vi "Yokogawa GS200 Coarse V ramp.vi"(5 "Time Interval (sec)":dbl=0.5 min=0.1 step=0.1, 6 "stop":bool, 7 "Sweep Time (H:M:S)":dbl=3600.0 format="%<%H:%M:%S>t", 8 "Mapping":bool, 9 "End Voltage (V)":dbl=1e-10 format="%.3e", 10 "Start Voltage (V)":dbl=1e-06 format="%.3e", 11 "Yokogawa GS200 Address":refnum<visa-resource-name>) -> (1 "Last Sent Value":dbl=1e-06 format="%.3e")   [LabVIEW 2020]
uses:
  Global Variables/Voltage Yokogawa Coarse.vi
panel:
  out "Iteration":i32
  out "Prepared Value":dbl=1e-06 format="%.3e"
  # "Add two extra sec for timing."
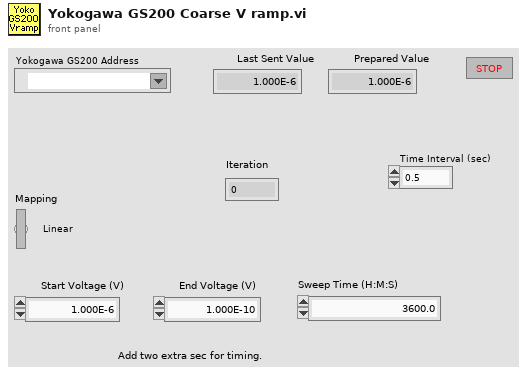
[diagram p1: front panel]
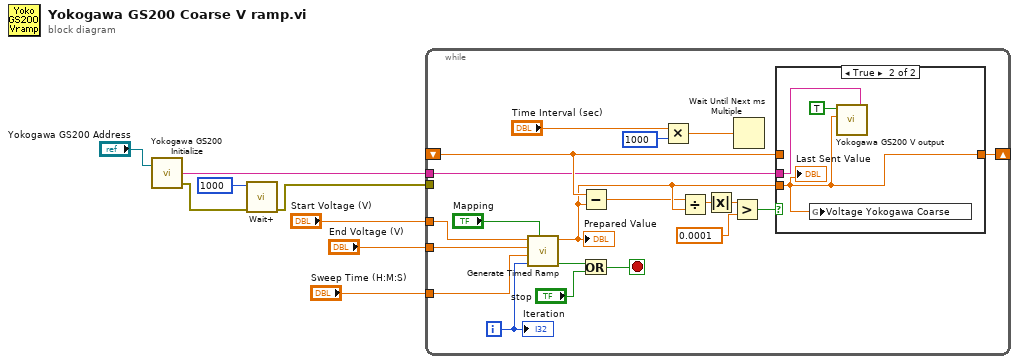
[diagram p0: block diagram]
diagram:
  n1 = call "Yokogawa GS200 Initialize.vi"("VISA resource name"="Yokogawa GS200 Address") -> ("Instrument ID String"=w8:string, "Error Out"=w4:errorcluster)  [unwired: 1 in, 1 out]
  n2 = call "Wait+.vi"("Error In"=w4, "milliseconds to wait"=u32 1000) -> ("Error Out"=w6:errorcluster)  [unwired: 4 in, 1 out]
  n3 = while {
    tunnel: "Start Voltage (V)" -> [w28]
    tunnel: "End Voltage (V)" -> [w27]
    tunnel: "Sweep Time (H:M:S)" -> [w26]
    shift-right: [w19] -> _
    shift-left: _ -> [w17]
    tunnel: w8 -> [w15]
    tunnel: w6 -> [_]
    i -> [w25]
    stop <- w23 stop-if-true
    n4 = call "Generate Timed Ramp.vi"("Log"="Mapping", "Point #"=w25, "Time (Hr:Min:Sec)"=w26, "Stop"=w27, "Start"=w28) -> ("Stop"=w22:bool, "Output"=w16:dbl)  [unwired: 2 out]
    "Prepared Value" <- w16
    n5 = Subtract(x=w17, y=w16) -> (x-y=w11:dbl)
    n6 = Or(x=w22, y="stop") -> (x .or. y?=w23:bool)
    n7 = Multiply(x="Time Interval (sec)", y=u32 1000 ("millisecond multiple")) -> (x*y=w13:dbl)
    n8 = Divide(x=w11, y=w16) -> (x/y=w9:dbl)
    n9 = Absolute Value(x=w9) -> (abs(x)=w10:dbl)
    n10 = Greater?(x=w10, y=0.0001) -> (0:w18:bool)
    n11 = Wait Until Next ms Multiple(millisecond multiple=w13) -> ()  [unwired: 1 out]
    n12 = case shown="True" w18 {
      tunnel: [w29 w30] -> w19
      tunnel: w17 -> [w29 _]
      tunnel: w16 -> [_ w30]
      tunnel: w15 -> [_ w31]
      frame False {
      }
      frame True {
        n13 = global write "Voltage Yokogawa Coarse.vi" "Voltage Yokogawa Coarse"(w30) -> ()
        n14 = call "Yokogawa GS200 V output.vi"("VISA resource name"=w31, "Voltage Level (0.0 V)"=w30, "Enable Output (T: Enable)"=TRUE) -> ()  [unwired: 2 in, 2 out]
        "Last Sent Value" <- w30
      }
    }
    "Iteration" <- w25
  }
